vi "generate 1 cycle.vi"(8 "error in (no error)":errorcluster caption="에러 입력(에러 없음)", 11 "Waveform Obj 입력":refnum<class "PWL_DW7802.lvclass">) -> (0 "error out":errorcluster caption="에러 출력", 2 "waveform":waveform(dbl), 3 "Waveform Obj 출력":refnum<class "PWL_DW7802.lvclass">)   [LabVIEW 2020, in "PWL_DW7802.lvclass"]
uses:
  PWL_DW7802.lvclass
  PWL/PWL.lvclass/PWL.ctl
  Waveform Obj/Waveform Obj.lvclass/Waveform Obj.ctl
  Waveform Gen/Waveform Gen.lvclass/Waveform Gen.ctl
  Sine Wave/Sine Wave.lvclass
  Square Wave/Square Wave.lvclass
  Waveform Obj/Accessors/Write sampling rate.vi
  Waveform Gen/Accessors/Write frequency.vi
  Waveform Gen/Accessors/Write scale.vi
  PWL/Accessors/Read waveform type.vi
  Waveform Obj/Accessors/Read sampling rate.vi
  Waveform Gen/Accessors/Read frequency.vi
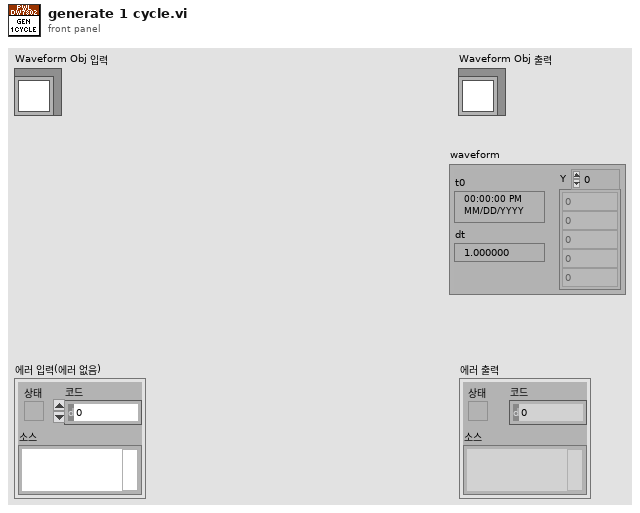
[diagram p1: front panel]
types:
  T1 = typedef "Waveform Gen.lvclass/waveform gen type.ctl" = enum16{"Sine", "Square", "Triangle", "Sawtooth", "Auto Track", "Auto Brake (Square)", "Auto Brake (Sine)", "PWL"}
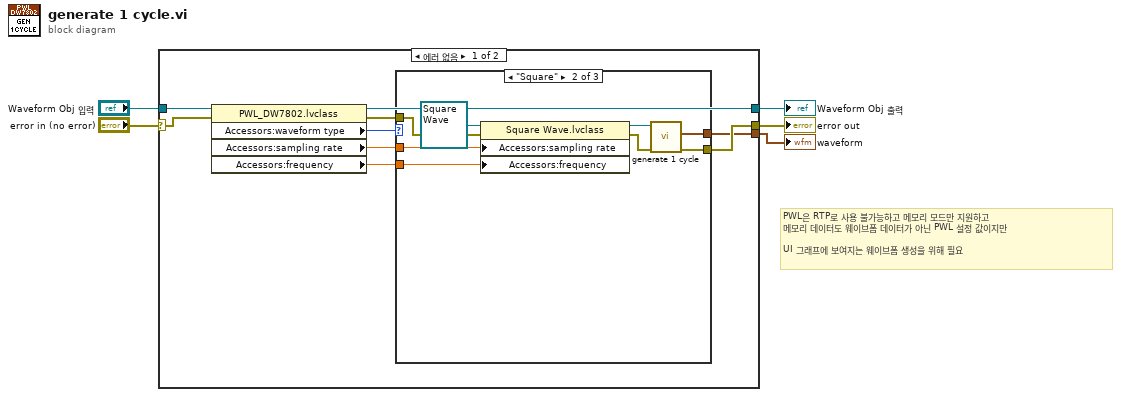
[diagram p0: block diagram]
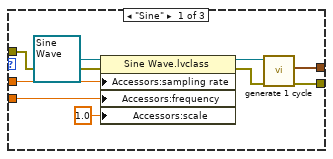
[diagram p2: hidden frame]
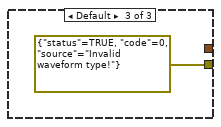
[diagram p3: hidden frame]
diagram:
  # "PWL은 RTP로 사용 불가능하고 메모리 모드만 지원하고\n메모리 데이터도 웨이브폼 데이터가 아닌 PWL 설정 값이지만\n\nUI 그래프에 보여지는 웨이브폼 생성을 위해 필요"
  n1 = case shown="에러 없음" "error in (no error)" {
    selector: "error in (no error)" -> [w12 w34]
    tunnel: [w9 w34] -> w5
    tunnel: [w13 w33] -> w4
    tunnel: "Waveform Obj 입력" -> [w14 w33]
    tunnel: [w6 _] -> w1
    frame No Error {
      n2 = property class="PWL_DW7802.lvclass"(reference=w14, error in=w12) -> (reference out=w13:refnum<class "PWL_DW7802.lvclass">, error out=w10:errorcluster, "Accessors:waveform type"=w11:T1, "Accessors:sampling rate"=w8:dbl, "Accessors:frequency"=w7:dbl)
      n3 = case shown="\"Square\"" w11 {
        tunnel: w10 -> [w19 w27 _]
        tunnel: [w17 w25 errorcluster {"status"=TRUE, "code"=0, "source"="Invalid waveform type!"} ("error out")] -> w9
        tunnel: w8 -> [w22 w30 _]
        tunnel: w7 -> [w21 w29 _]
        tunnel: [w16 w24 _] -> w6
        frame "Sine" {
          n4 = property class="Sine Wave.lvclass"(reference=refnum<class "Sine Wave.lvclass"> refnum ("Sine Wave.lvclass"), error in=w19, "Accessors:sampling rate"=w22, "Accessors:frequency"=w21, "Accessors:scale"=1.0 ("scale")) -> (reference out=w20:refnum<class "Sine Wave.lvclass">, error out=w18:errorcluster)
          n5 = call-dynamic "generate 1 cycle.vi"("error in (no error)"=w18, "Sine Wave 입력"=w20) -> ("error out"=w17:errorcluster, "waveform"=w16:waveform(dbl))  [unwired: 7 in, 1 out]
        }
        frame "Square" {
          n6 = property class="Square Wave.lvclass"(reference=refnum<class "Square Wave.lvclass"> refnum ("Square Wave.lvclass"), error in=w27, "Accessors:sampling rate"=w30, "Accessors:frequency"=w29) -> (reference out=w28:refnum<class "Square Wave.lvclass">, error out=w26:errorcluster)
          n7 = call-dynamic "generate 1 cycle.vi"("error in (no error)"=w26, "Square Wave 입력"=w28) -> ("error out"=w25:errorcluster, "waveform"=w24:waveform(dbl))  [unwired: 7 in, 1 out]
        }
        frame Default {
        }
      }
    }
    frame Error {
    }
  }
  "error out" <- w5
  "Waveform Obj 출력" <- w4
  "waveform" <- w1
